vi "Bandpass Signal Generator.vi"(3 "sampling info":cluster{"Fs":dbl, "#s":dbl}={"Fs"=60000.0, "#s"=400.0} {"Fs" format="%.2p"}, 4 "Bandwidth":dbl=1000.0 format="%#_6p", 5 "Center Frequency":dbl=5000.0 format="%#_6p") -> (1 "Bandpass Signal":waveform(dbl))   [LabVIEW 2009]
uses:
  <vilib>/measure/maspectr.llb/FFT Power Spectrum for 1 Chan.vi
  <vilib>/Analysis/3filter.llb/Butterworth Filter (DBL).vi
  <vilib>/measure/NI_MAPro.lvlib
  <vilib>/Analysis/NI_AALBase.lvlib
panel:
  out "Waveform Graph 2":cluster{"f0":dbl, "df":dbl, "magnitude":dbl[]}[](graph)
  out "Waveform Graph":waveform(dbl)[](graph)
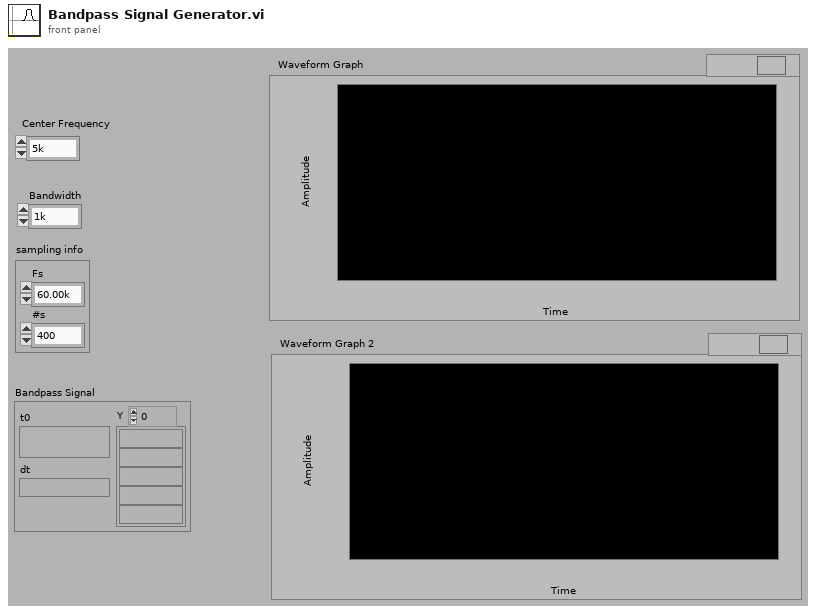
[diagram p1: front panel]
types:
  T1 = enum32{"Lowpass", "Highpass", "Bandpass", "Bandstop"}
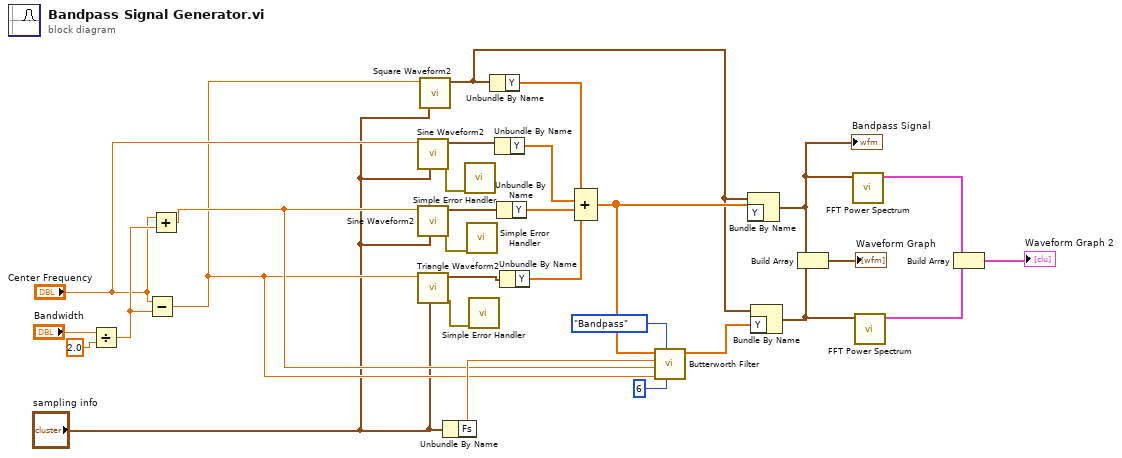
[diagram p0: block diagram]
diagram:
  n1 = Divide(x="Bandwidth", y=2.0) -> (x/y=w27:dbl)
  n2 = Subtract(x="Center Frequency", y=w27) -> (x-y=w5:dbl)
  n3 = Add(x="Center Frequency", y=w27) -> (x+y=w21:dbl)
  n4 = call "Sine Waveform2.vi"("sampling info"="sampling info", "frequency"="Center Frequency") -> ("error out"=w9:errorcluster, "signal out"=w18:waveform(dbl))  [unwired: 8 in]
  n5 = call "Sine Waveform2.vi"("sampling info"="sampling info", "frequency"=w21) -> ("error out"=w10:errorcluster, "signal out"=w25:waveform(dbl))  [unwired: 8 in]
  n6 = call "Triangle Waveform2.vi"("sampling info"="sampling info", "frequency"=w5) -> ("error out"=w11:errorcluster, "signal out"=w8:waveform(dbl))  [unwired: 8 in]
  n7 = call "Square Waveform2.vi"("sampling info"="sampling info", "frequency"=w5) -> ("signal out"=w3:waveform(dbl))  [unwired: 8 in, 1 out]
  n8 = Unbundle By Name("sampling info") -> ("Fs"=w22:dbl)
  n9 = call <vilib>:"Simple Error Handler.vi"("error in (no error)"=w9) -> ()  [unwired: 4 in, 5 out]
  n10 = call <vilib>:"Simple Error Handler.vi"("error in (no error)"=w10) -> ()  [unwired: 4 in, 5 out]
  n11 = call <vilib>:"Simple Error Handler.vi"("error in (no error)"=w11) -> ()  [unwired: 4 in, 5 out]
  n12 = Unbundle By Name(w3) -> ("Y"=w2:dbl[])
  n13 = Unbundle By Name(w18) -> ("Y"=w1:dbl[])
  n14 = Unbundle By Name(w25) -> ("Y"=w24:dbl[])
  n15 = Unbundle By Name(w8) -> ("Y"=w23:dbl[])
  n16 = Compound Arithmetic op=ADD(w2, w1, w24, w23) -> (w17:dbl[])
  n17 = call-poly <vilib>:"Butterworth Filter.vi"("order"=6, "filter type"=T1."Bandpass", "low cutoff freq: fl"=w5, "high cutoff freq: fh"=w21, "sampling freq: fs"=w22, "X"=w17) -> ("Filtered X"=w16:dbl[])  [unwired: 2 in, 1 out]
  n18 = Bundle By Name(cluster=w3, "Y"=w17) -> (w7:waveform(dbl))
  "Bandpass Signal" <- w7
  n19 = Bundle By Name(cluster=w3, "Y"=w16) -> (w12:waveform(dbl))
  n20 = Build Array(w7, w12) -> (→"Waveform Graph":waveform(dbl)[])
  n21 = call-poly <vilib>:"FFT Power Spectrum.vi"("time signal"=w7) -> ("power spectrum"=w15:cluster{"f0":dbl, "df":dbl, "magnitude":dbl[]})  [unwired: 7 in, 3 out]
  n22 = call-poly <vilib>:"FFT Power Spectrum.vi"("time signal"=w12) -> ("power spectrum"=w14:cluster{"f0":dbl, "df":dbl, "magnitude":dbl[]})  [unwired: 7 in, 3 out]
  n23 = Build Array(w15, w14) -> (→"Waveform Graph 2":cluster{"f0":dbl, "df":dbl, "magnitude":dbl[]}[])
